vi "CheckLevels.vi"(6 "op states match":bool, 8 "error in (no error)":errorcluster, 9 "value":dbl, 10 "rule":T3, 11 "cache in":T1) -> (0 "error out":errorcluster, 1 "update trend":bool, 2 "update file":bool, 3 "cache out":T1)   [LabVIEW 2017, in "TrendAlarm.lvlib"]
uses:
  <vilib>/addons/InsightCM/Devices/Shared/Common/TrendAlarm/TrendAlarm.lvlib
  <vilib>/addons/InsightCM/MessageBus/Base/controls/TrendAlarmRule.ctl
  <vilib>/addons/InsightCM/MessageBus/Base/controls/TrendAlarmLevel.ctl
  <vilib>/addons/InsightCM/MessageBus/Base/controls/AlarmAction.ctl
  <vilib>/addons/InsightCM/MessageBus/Base/controls/KeyValuePair.ctl
  <vilib>/addons/InsightCM/Devices/Shared/Common/TrendAlarm/controls/TransitionCache.ctl
  <vilib>/addons/InsightCM/MessageBus/Base/controls/TrendAlarmTransition.ctl
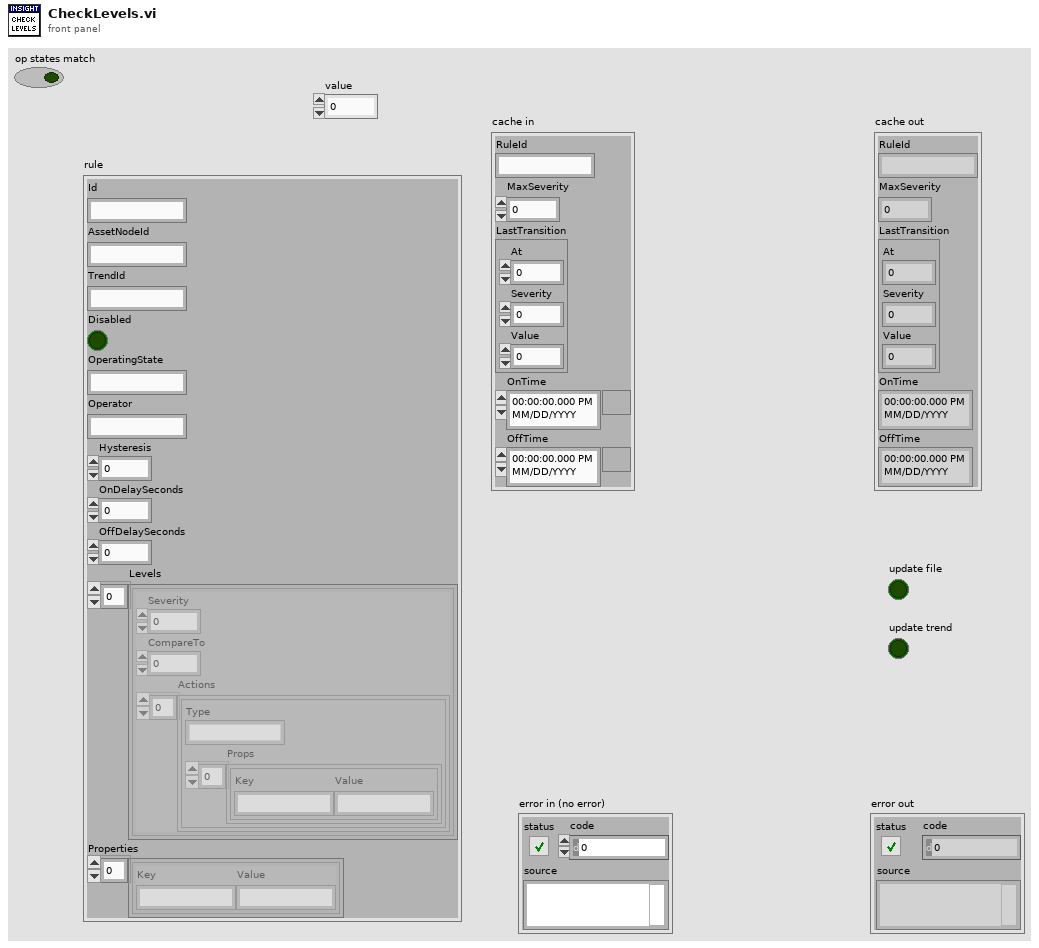
[diagram p1: front panel]
types:
  T1 = typedef "TrendAlarm.lvlib/TransitionCache.ctl" = cluster{"RuleId":string, "MaxSeverity":i32, "LastTransition":T2, "OnTime":timestamp, "OffTime":timestamp}
  T2 = typedef "TrendAlarmTransition.ctl" = cluster{"At":i64, "Severity":i32, "Value":dbl}
  T3 = typedef "TrendAlarmRule.ctl" = cluster{"Id":string, "AssetNodeId":string, "TrendId":string, "Disabled":bool, "OperatingState":string, "Operator":string, "Hysteresis":dbl, "OnDelaySeconds":dbl, "OffDelaySeconds":dbl, "Levels":T4[], "Properties":T6[]}
  T4 = typedef "TrendAlarmLevel.ctl" = cluster{"Severity":i32, "CompareTo":dbl, "Actions":T5[]}
  T5 = typedef "AlarmAction.ctl" = cluster{"Type":string, "Props":T6[]}
  T6 = typedef "KeyValuePair.ctl" = cluster{"Key":string, "Value":string}
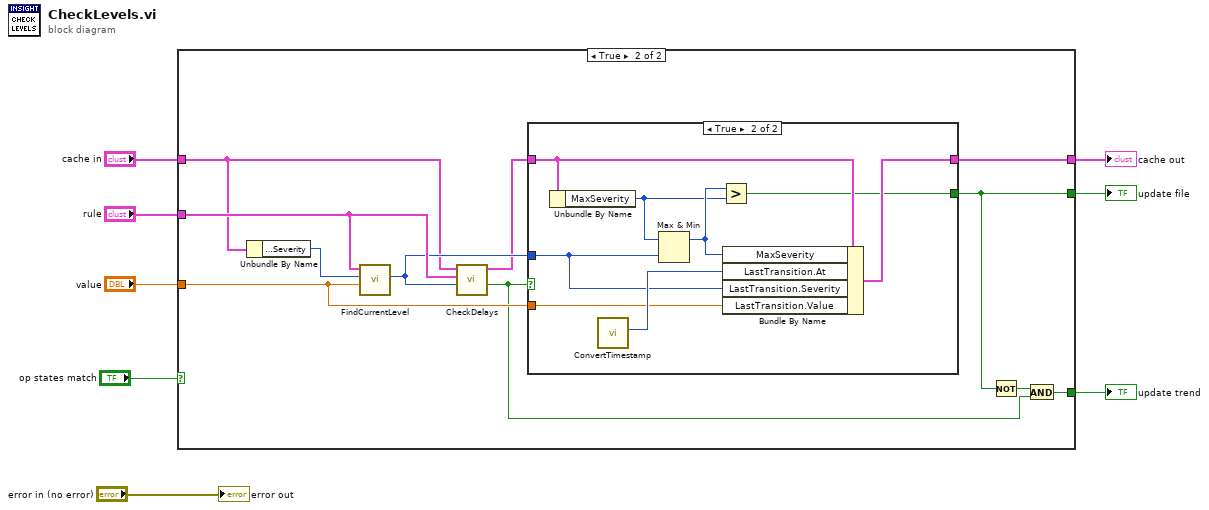
[diagram p0: block diagram]
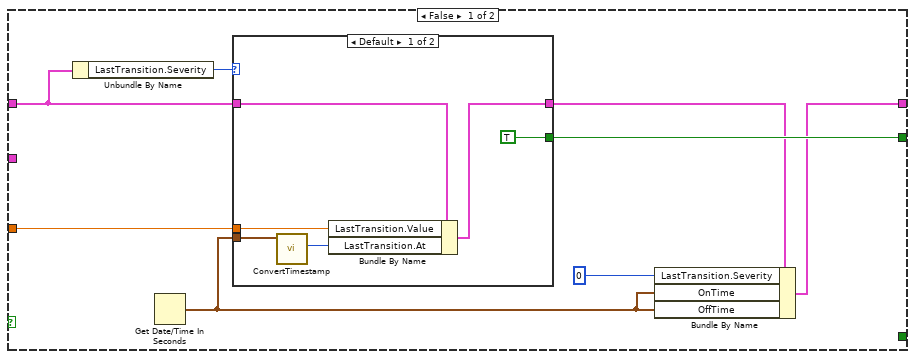
[diagram p2: hidden frame]
diagram:
  n1 = case shown="True" "op states match" {
    tunnel: "rule" -> [_ w34]
    tunnel: "value" -> [w9 w31]
    tunnel: "cache in" -> [w14 w30]
    tunnel: [w12 w28] -> w5
    tunnel: [w15 w27] -> w3
    tunnel: [_ w24] -> w2
    frame False {
      n2 = Unbundle By Name(w14) -> ("LastTransition.Severity"=w16:i32)
      n3 = Get Date/Time In Seconds() -> (seconds since 1Jan1904=w10:timestamp)
      n4 = case shown="Default" w16 {
        tunnel: [TRUE _] -> w15
        tunnel: w14 -> [w21 w23]
        tunnel: [w20 w23] -> w13
        tunnel: w10 -> [w19 _]
        tunnel: w9 -> [w18 _]
        frame Default {
          n5 = call <vilib>:"ConvertTimestamp.vi"("Time Stamp"=w19) -> ("Timestamp out"=w17:i64)  [unwired: 10 in]
          n6 = Bundle By Name(cluster=w21, "LastTransition.Value"=w18, "LastTransition.At"=w17) -> (w20:T1)
        }
        frame 0 {
        }
      }
      n7 = Bundle By Name(cluster=w13, "LastTransition.Severity"=0, "OnTime"=w10, "OffTime"=w10) -> (w12:T1)
    }
    frame True {
      n8 = Unbundle By Name(w30) -> ("LastTransition.Severity"=w33:i32)
      n9 = call <vilib>:"FindCurrentLevel.vi"("value"=w31, "latched severity"=w33, "rule"=w34) -> ("severity out"=w32:i32)  [unwired: 8 in]
      n10 = call <vilib>:"CheckDelays.vi"("current level"=w32, "rule"=w34, "cache in"=w30) -> ("update"=w25:bool, "cache out"=w29:T1)  [unwired: 7 in]
      n11 = case shown="True" w25 {
        tunnel: w29 -> [w35 w40]
        tunnel: w32 -> [_ w39]
        tunnel: w31 -> [_ w42]
        tunnel: [w35 w41] -> w28
        tunnel: [_ w37] -> w27
        frame False {
        }
        frame True {
          n12 = Unbundle By Name(w40) -> ("MaxSeverity"=w36:i32)
          n13 = call <vilib>:"ConvertTimestamp.vi"() -> ("Timestamp out"=w43:i64)  [unwired: 11 in]
          n14 = Max & Min(x=w36, y=w39) -> (max(x,y)=w38:i32)  [unwired: 1 out]
          n15 = Greater?(x=w38, y=w36) -> (0:w37:bool)
          n16 = Bundle By Name(cluster=w40, "MaxSeverity"=w38, "LastTransition.At"=w43, "LastTransition.Severity"=w39, "LastTransition.Value"=w42) -> (w41:T1)
        }
      }
      n17 = Not(x=w27) -> (.not. x?=w26:bool)
      n18 = And(x=w26, y=w25) -> (x .and. y?=w24:bool)
    }
  }
  "cache out" <- w5
  "update trend" <- w2
  "update file" <- w3
  "error out" <- "error in (no error)"
